vi "writeToTable.vi"(8 "error in (no error)":errorcluster, 10 "Item Names":string[][](array[string]), 11 "GoalUserInterface in":refnum<class "GoalUserInterface.lvclass">) -> (0 "error out":errorcluster, 3 "GoalUserInterface out":refnum<class "GoalUserInterface.lvclass">)   [LabVIEW 2018, in "GoalUserInterface.lvclass"]
uses:
  GoalUserInterface.lvclass
  GoalUserInterface.lvclass/GoalUserInterface.ctl
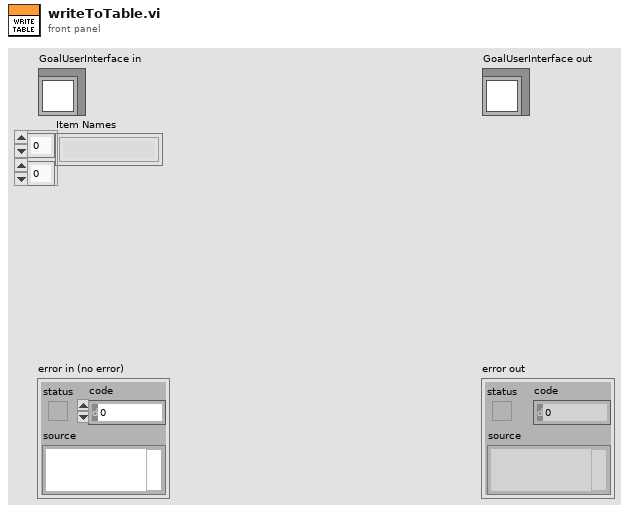
[diagram p1: front panel]
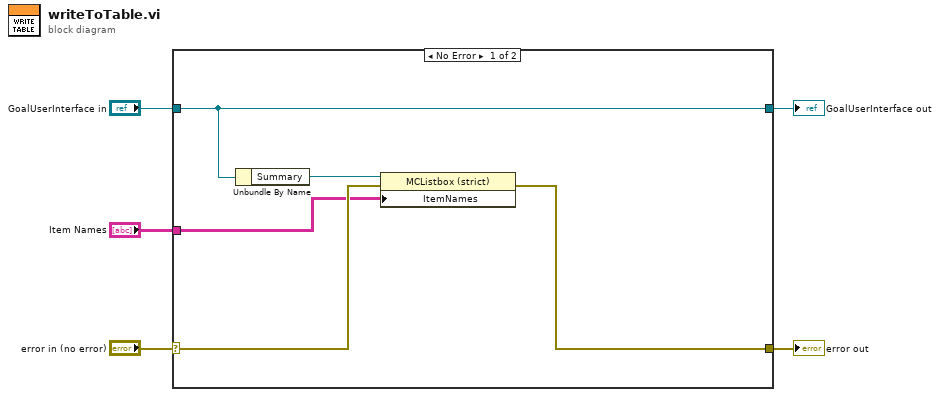
[diagram p0: block diagram]
diagram:
  n1 = case shown="No Error" "error in (no error)" {
    selector: "error in (no error)" -> [w9 w12]
    tunnel: [w8 w12] -> w4
    tunnel: [w6 w11] -> w2
    tunnel: "GoalUserInterface in" -> [w6 w11]
    tunnel: "Item Names" -> [w7 _]
    frame No Error {
      n2 = Unbundle By Name(w6) -> ("Summary"=w10:refnum<vi>)
      n3 = property class="MCListbox (strict)"(reference=w10, error in=w9, "ItemNames"=w7) -> (error out=w8:errorcluster)  [unwired: 1 out]
    }
    frame Error {
    }
  }
  "error out" <- w4
  "GoalUserInterface out" <- w2
